vi "Write CustomNikon.vi"(8 "error in (no error)":errorcluster, 10 "CustomNikon":string, 11 "Nikon in":refnum<class "Nikon.lvclass">) -> (0 "error out":errorcluster, 3 "Nikon out":refnum<class "Nikon.lvclass">)   [LabVIEW 2021, in "Nikon.lvclass"]
uses:
  Nikon.lvclass
  Nikon.lvclass/Nikon.ctl
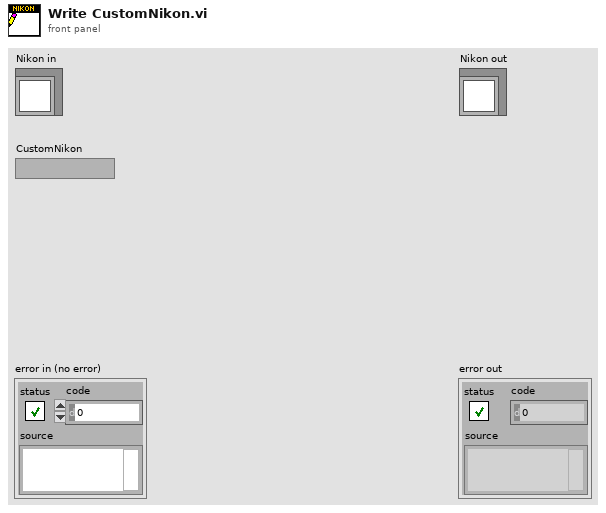
[diagram p1: front panel]
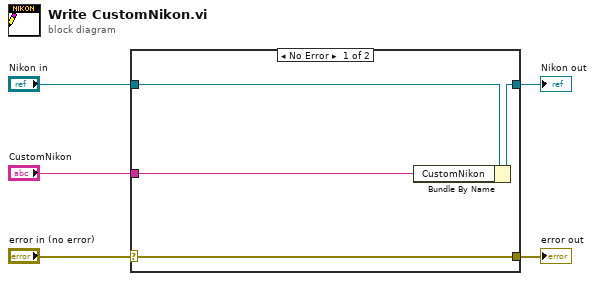
[diagram p0: block diagram]
diagram:
  n1 = case shown="No Error" "error in (no error)" {
    selector: "error in (no error)" -> [w9 w10]
    tunnel: [w9 w10] -> w4
    tunnel: [w7 w11] -> w2
    tunnel: "Nikon in" -> [w8 w11]
    tunnel: "CustomNikon" -> [w6 _]
    frame No Error {
      n2 = Bundle By Name(cluster=w8, "CustomNikon"=w6) -> (w7:refnum<class "Nikon.lvclass">)
    }
    frame Error {
    }
  }
  "error out" <- w4
  "Nikon out" <- w2
